vi "Update Processing Metrics.vi"(8 "error in (no error)":errorcluster, 9 "Peak Output":dbl, 10 "System Throughput":dbl, 11 "Application Manager in":refnum<class "Application Manager.lvclass">) -> (0 "error out":errorcluster, 3 "Application Manager out":refnum<class "Application Manager.lvclass">)   [LabVIEW 2020, in "Application Manager.lvlib" / "Application Manager.lvclass"]
uses:
  Application Manager.lvclass
  Application Manager.lvclass/Application Manager.ctl
  UI/UI Root/UI Root Messages/Update Processing Metrics Msg/Update Processing Metrics Msg.lvclass/Update Processing Metrics Msg.ctl
  <vilib>/ActorFramework/Message Enqueuer/Message Enqueuer.lvclass/Message Enqueuer.ctl
  <vilib>/ActorFramework/Message Enqueuer/Enqueue.vi
  UI/UI Root/UI Root Messages/Update Processing Metrics Msg/Update Processing Metrics Msg.lvclass
  C:/Program Files/National Instruments/LabVIEW 2025/vi.lib/ActorFramework/Message/Message.lvclass
  <vilib>/ActorFramework/Message Priority Queue/Priority Enqueue.vi
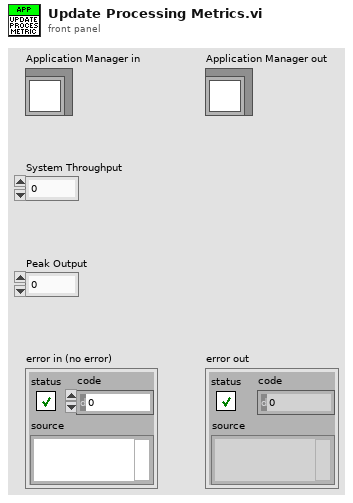
[diagram p1: front panel]
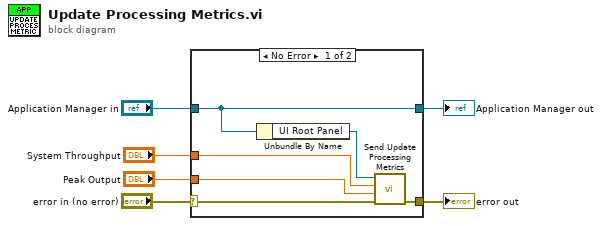
[diagram p0: block diagram]
diagram:
  n1 = case shown="No Error" "error in (no error)" {
    selector: "error in (no error)" -> [w10 w14]
    tunnel: [w9 w14] -> w5
    tunnel: [w12 w13] -> w3
    tunnel: "Application Manager in" -> [w12 w13]
    tunnel: "System Throughput" -> [w8 _]
    tunnel: "Peak Output" -> [w7 _]
    frame No Error {
      n2 = Unbundle By Name(w12) -> ("UI Root Panel"=w11:refnum<class "Message Enqueuer.lvclass">)
      n3 = call "Send Update Processing Metrics.vi"("error in (no error)"=w10, "Peak Output"=w7, "System Throughput"=w8, "Message Enqueuer"=w11) -> ("error out"=w9:errorcluster)  [unwired: 6 in, 1 out]
    }
    frame Error {
    }
  }
  "error out" <- w5
  "Application Manager out" <- w3
